vi "measure_dc2400_lxy.vi"() -> ()   [LabVIEW 2019, in "SubVI.lvlib"]
uses:
  SubVI.lvlib
  config.ctl
  <vilib>/NI/Modbus Library/API/Master/Modbus Master.lvclass
  initialize.ctl
  Instrument.ctl
  Instrument Type.ctl
  C:/Users/star/Desktop/measrue/lib/QDInstrument.dll
  lib/QDInstrument.dll
  335 state.ctl
  <vilib>/Analysis/baseanly.llb/Mean (DBL).vi
  lib/Keithley 24XX/Public/Data/Read (Single Point).vi
  Get value.lvlib
  <vilib>/Analysis/NI_AALBase.lvlib
  lib/Keithley 24XX/Keithley 24XX.lvlib
panel:
  out "输出数组":string[](array[string])
  in  "输入簇":T1={"initialize"=enum."SR830", "6221"={"6221 Resource"="GPIB0::24::INSTR", "Delta status"=FALSE, "电流"=0.0}, "SR830+6221"={"source"=0, "阻抗"=0.0, "量程入 4"=0, "量程入 3"=0, "量程入 2"=0, "量程入 1"=0, "SR830 2"=FALSE, "SR830 3"=FALSE, "SR830 4"=FALSE, "SR830 1"=FALSE, "VISA 1"="", "VISA 2"="", "VISA 3"="", "VISA 4"="", "Reserve 1"=0, "Reserve 2"=-1, "Reserve 3"=-1, "Reserve 4"=-1, "量程"=enum."量程每次测量会判定"}, "2400"={"2400"=FALSE, "VISA"=""}, "ch"={"ch"=[], "current"=[], "change?"=[], "holding current\nwhen change ch?"=FALSE}, "Instrument"={"335 Resource"="GPIB0::24::INSTR", "Input (0:A)"=0, "Instrument Type"=enum."SVSM", "quantum design"=refnum, "Heater Output (1:1)"=1, "semaphore"=refnum, "TCP master instance"=refnum, "335 Status"=refnum, "M24C Resource"="GPIB0::24::INSTR", "4G supply"="GPIB0::24::INSTR", "Temp Status 24C"=refnum, "4g supply status"=refnum, "Temp"=refnum}, "Aborting"=refnum, "数据文件"=refnum} {"Instrument"."Input (0:A)" items=["A", "B"]; "Instrument"."Heater Output (1:1)" items=["1"=1, "2"=2]; "SR830+6221"."Reserve 4" items=["Auto Reserve"=-1, "High Reserve"=0, "Normal"=1, "Low Noise"=2]; "SR830+6221"."Reserve 3" items=["Auto Reserve"=-1, "High Reserve"=0, "Normal"=1, "Low Noise"=2]; "SR830+6221"."Reserve 2" items=["Auto Reserve"=-1, "High Reserve"=0, "Normal"=1, "Low Noise"=2]; "SR830+6221"."Reserve 1" items=["量程每次测量会判定", "量程不变为设定值"]; "SR830+6221"."source" items=["SR830 1", "SR830 2", "SR830 3", "SR830 4"]}
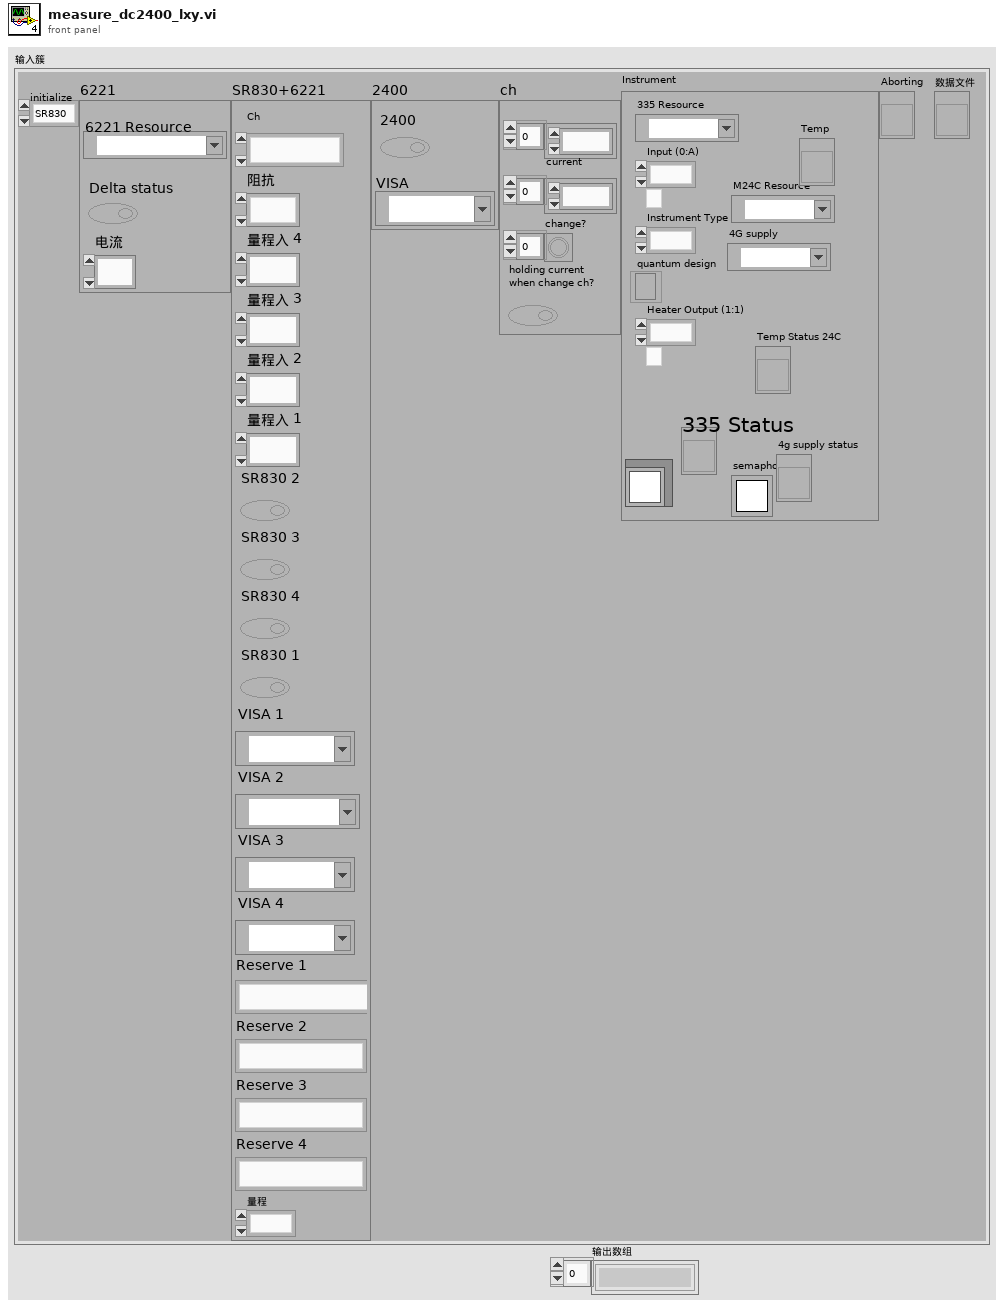
[diagram p1: front panel]
types:
  T1 = typedef "config.ctl" = cluster{"initialize":T2, "6221":cluster{"6221 Resource":refnum<visa-resource-name>, "Delta status":bool, "电流":dbl}, "SR830+6221":cluster{"source":u16, "阻抗":dbl, "量程入 4":i32, "量程入 3":i32, "量程入 2":i32, "量程入 1":i32, "SR830 2":bool, "SR830 3":bool, "SR830 4":bool, "SR830 1":bool, "VISA 1":refnum<visa-resource-name>, "VISA 2":refnum<visa-resource-name>, "VISA 3":refnum<visa-resource-name>, "VISA 4":refnum<visa-resource-name>, "Reserve 1":i16, "Reserve 2":i16, "Reserve 3":i16, "Reserve 4":i16, "量程":enum16{"量程每次测量会判定", "量程不变为设定值"}}, "2400":cluster{"2400":bool, "VISA":refnum<visa-resource-name>}, "ch":cluster{"ch":i32[], "current":dbl[], "change?":bool[], "holding current\nwhen change ch?":bool}, "Instrument":T3, "Aborting":refnum<vi>, "数据文件":refnum<vi>}
  T2 = typedef "initialize.ctl" = enum16{"SR830", "keithley6221-SR830", "Delta", "Delta-tunnelling", "keithley6221-2182-DC"}
  T3 = typedef "Instrument.ctl" = cluster{"335 Resource":refnum<visa-resource-name>, "Input (0:A)":u16, "Instrument Type":T4, "quantum design":refnum<k24>, "Heater Output (1:1)":u16, "semaphore":T5, "TCP master instance":refnum<class "Modbus Master.lvclass">, "335 Status":refnum<vi>, "M24C Resource":refnum<visa-resource-name>, "4G supply":refnum<visa-resource-name>, "Temp Status 24C":refnum<vi>, "4g supply status":refnum<vi>, "Temp":refnum<vi>}
  T4 = typedef "Instrument Type.ctl" = enum16{"PPMS", "VersaLab", "DynaCool", "SVSM", "PPMS-Rotate", "Lakeshore335", "9T mag"}
  T5 = typedef "Semaphore RefNum" = refnum<k1>
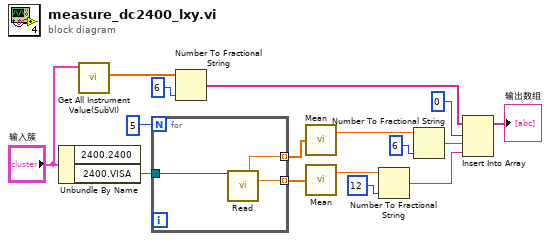
[diagram p0: block diagram]
diagram:
  n1 = Unbundle By Name("输入簇") -> ("2400.VISA"=w3:refnum<visa-resource-name>)  [unwired: 1 out]
  n2 = call "Get All Instrument Value(SubVI).vi"("输出簇 2"="输入簇") -> ("数组"=w15:dbl[])  [unwired: 10 in]
  n3 = for {
    N: 5 -> [_]
    tunnel: [w19] -> w8 mode=indexing
    tunnel: [w18] -> w7 mode=indexing
    tunnel: w3 -> [w17]
    n4 = call-poly "Read.vi"("VISA resource name"=w17) -> ("Voltage"=w19:sgl, "Current"=w18:sgl)  [unwired: 8 in, 5 out]
  }
  n5 = Number To Fractional String(number=w15, precision (6)=i16 6 ("精度(6)")) -> (F-format string=w14:string[])  [unwired: 2 in]
  n6 = call-poly <vilib>:"Mean.vi"("X"=w8) -> ("mean"=w11:dbl)  [unwired: 1 out]
  n7 = call-poly <vilib>:"Mean.vi"("X"=w7) -> ("mean"=w6:dbl)  [unwired: 1 out]
  n8 = Number To Fractional String(number=w6, precision (6)=i16 12 ("精度(6)")) -> (F-format string=w5:string)  [unwired: 2 in]
  n9 = Number To Fractional String(number=w11, precision (6)=i16 6 ("精度(6)")) -> (F-format string=w10:string)  [unwired: 2 in]
  n10 = Insert Into Array(array=w14, index=0 ("索引"), new element #1=w10, new element #2=w5) -> (→"输出数组":string[])
